vi "Turn_off_eclipse.vi"(8 "error in (no error)":errorcluster, 9 "Boolean":bool, 10 "Numeric":i32, 11 "VISA Refnum in":refnum<visa-resource-name>) -> (0 "error out":errorcluster, 3 "VISA Refnum out":refnum<visa-resource-name>)   [LabVIEW 2015]
uses:
  utilities/Test_Code/Global 5.vi
  <instrlib>/Agilent N6700 Series/Agilent N6700 Series.lvlib
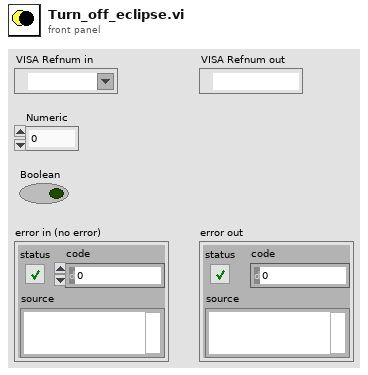
[diagram p1: front panel]
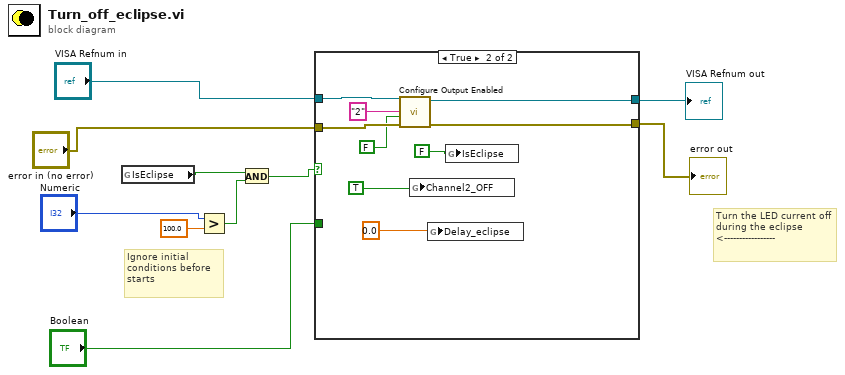
[diagram p0: block diagram]
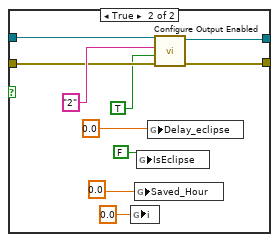
[diagram p3: hidden frame]
diagram:
  # "Ignore initial conditions before starts"
  # "Turn the LED current off during the eclipse \n<-----------------"
  n1 = global read "Global 5.vi" "IsEclipse"() -> (w8:bool)
  n2 = Greater?(x="Numeric", y=100.0) -> (0:w4:bool)
  n3 = And(x=w8, y=w4) -> (x .and. y?=w1:bool)
  n4 = case shown="True" w1 {
    tunnel: "VISA Refnum in" -> [w14 w35]
    tunnel: "error in (no error)" -> [w15 w34]
    tunnel: [w12 w32] -> w7
    tunnel: [w13 w31] -> w6
    tunnel: "Boolean" -> [w11 _]
    frame False {
      n5 = case shown="False" w11 {
        tunnel: w14 -> [w16 w22]
        tunnel: w15 -> [w17 w26]
        tunnel: [w17 w24] -> w12
        tunnel: [w16 w23] -> w13
        frame False {
        }
        frame True {
          n6 = global write "Global 5.vi" "i"(0.0 ("i")) -> ()
          n7 = global write "Global 5.vi" "Saved_Hour"(0.0 ("Numeric")) -> ()
          n8 = global write "Global 5.vi" "IsEclipse"(FALSE ("Boolean")) -> ()
          n9 = global write "Global 5.vi" "Delay_eclipse"(0.0 ("Delay_eclipse")) -> ()
          n10 = call <instrlib>:"Configure Output Enabled.vi"("error in (no error)"=w26, "Enable Output (False)"=TRUE, "Channel Name (1)"="2", "VISA resource name"=w22) -> ("error out"=w24:errorcluster, "VISA resource name out"=w23:refnum<visa-resource-name>)  [unwired: 6 in]
        }
      }
    }
    frame True {
      n11 = call <instrlib>:"Configure Output Enabled.vi"("error in (no error)"=w34, "Enable Output (False)"=FALSE, "Channel Name (1)"="2", "VISA resource name"=w35) -> ("error out"=w32:errorcluster, "VISA resource name out"=w31:refnum<visa-resource-name>)  [unwired: 6 in]
      n12 = global write "Global 5.vi" "Channel2_OFF"(TRUE ("Channel2")) -> ()
      n13 = global write "Global 5.vi" "Delay_eclipse"(0.0 ("Delay_eclipse")) -> ()
      n14 = global write "Global 5.vi" "IsEclipse"(FALSE ("Boolean")) -> ()
    }
  }
  "error out" <- w7
  "VISA Refnum out" <- w6
